vi "T_RH_P.vi"(0 "VISA in":refnum<visa-resource-name>="LuftWS", 5 "WS_Commands":enum16{"OpenWS", "ReadTRHP", "CloseWS"}(ring)=enum."ReadTRHP", 7 "wait (ms)":u32=50, 11 "Error In":errorcluster) -> (4 "VISA out":refnum<visa-resource-name>="LuftWS", 6 "TRHP":T1={"Temp"=27.834401709401718, "RelH"=23.501221001221, "Press"=837.9120879120879, "AbH"=6.333943833943834}, 15 "Error Out":errorcluster)   [LabVIEW 2012]
uses:
  <vilib>/Instr/_visa.llb/VISA Configure Serial Port (Instr).vi
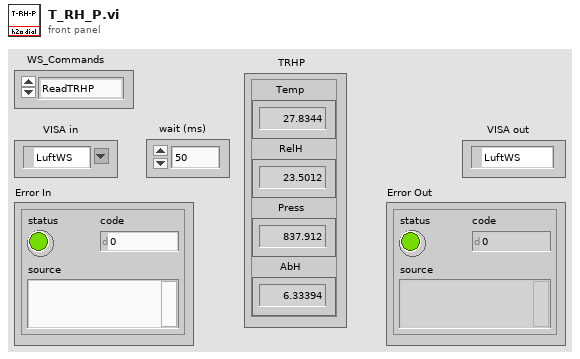
[diagram p1: front panel]
types:
  T1 = cluster{"Temp":dbl, "RelH":dbl, "Press":dbl, "AbH":dbl}
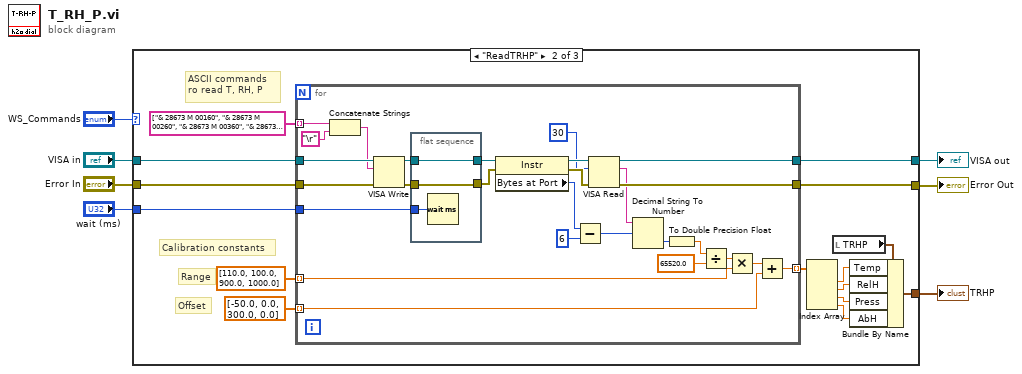
[diagram p0: block diagram]
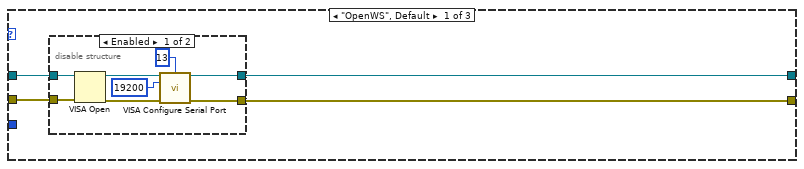
[diagram p2: hidden frame]
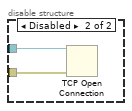
[diagram p3: hidden frame]
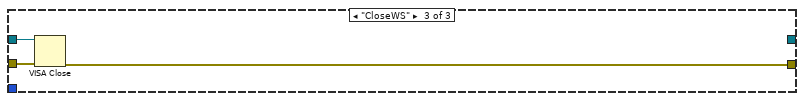
[diagram p4: hidden frame]
diagram:
  n1 = case shown="\"ReadTRHP\"" "WS_Commands" {
    tunnel: "VISA in" -> [w11 w36 w69]
    tunnel: "Error In" -> [w10 w35 w68]
    tunnel: [w9 w33 _] -> w3
    tunnel: [w8 w32 w67] -> w2
    tunnel: "wait (ms)" -> [_ w34 _]
    tunnel: [_ w30 _] -> w1
    frame "OpenWS", Default {
      n2 = disable-structure shown="Enabled" {
        disable-tunnel: w11 -> [w17 w21]
        disable-tunnel: w10 -> [w16 w20]
        disable-tunnel: [w14 _] -> w9
        disable-tunnel: [w13 _] -> w8
        frame Enabled {
          n3 = VISA Open(error in (no error)=w16, VISA resource name=w17) -> (VISA resource name=w19:refnum<visa-resource-name>, error out=w15:errorcluster)  [unwired: 3 in]
          n4 = call-poly "VISA Configure Serial Port"("VISA resource name"=w19, "termination char\n(0xA = '\\n' = LF)"=u8 13 ("termination char\n(0xA = '\\n' = LF)"), "baud rate (9600)"=u32 19200, "error in (no error)"=w15) -> ("VISA resource name out"=w14:refnum<visa-resource-name>, "error out"=w13:errorcluster)  [unwired: 10 in]
        }
        frame Disabled {
          n5 = TCP Open Connection(address=w21, error in (no error)=w20) -> ()  [unwired: 3 in, 2 out]
        }
      }
    }
    frame "ReadTRHP" {
      # "Offset"
      # "Range"
      # "Calibration constants"
      # "ASCII commands\nro read T, RH, P"
      n6 = for {
        tunnel: w36 -> [w63]
        tunnel: w35 -> [w62]
        tunnel: w34 -> [w58]
        tunnel: [w53] -> w33
        tunnel: [w52] -> w32
        tunnel: [w43] -> w26 mode=indexing
        tunnel: string[] ["& 28673 M 00160", "& 28673 M 00260", "& 28673 M 00360", "& 28673 M 00270"] -> [w40] mode=indexing
        tunnel: dbl[] [110.0, 100.0, 900.0, 1000.0] -> [w39] mode=indexing
        tunnel: dbl[] [-50.0, 0.0, 300.0, 0.0] -> [w38] mode=indexing
        n7 = Concatenate Strings(w40, "\r") -> (w59:string)
        n8 = VISA Write(VISA resource name=w63, write buffer=w59, error in (no error)=w62) -> (VISA resource name out=w60:refnum<visa-resource-name>, error out=w61:errorcluster)  [unwired: 1 out]
        n9 = flat-sequence {
          tunnel: [w66] -> w55
          tunnel: w60 -> [w66]
          tunnel: [w65] -> w54
          tunnel: w61 -> [w65]
          tunnel: w58 -> [w64]
          frame #0 {
            n10 = Wait (ms)(milliseconds to wait=w64) -> ()  [unwired: 1 out]
          }
        }
        n11 = property class="Instr"(reference=w55, error in=w54) -> (reference out=w56:refnum<visa-resource-name>, error out=w57:errorcluster, "Bytes at Port"=w51:u32)
        n12 = Subtract(x=w51, y=u32 6) -> (x-y=w48:u32)
        n13 = VISA Read(VISA resource name=w56, byte count=u32 30, error in (no error)=w57) -> (VISA resource name out=w53:refnum<visa-resource-name>, read buffer=w49:string, error out=w52:errorcluster)  [unwired: 1 out]
        n14 = Decimal String To Number(string=w49, offset=w48) -> (number=w47:i32)  [unwired: 1 in, 1 out]
        n15 = To Double Precision Float(number=w47) -> (double precision float=w46:dbl)
        n16 = Divide(x=w46, y=65520.0) -> (x/y=w45:dbl)
        n17 = Multiply(x=w45, y=w39) -> (x*y=w44:dbl)
        n18 = Add(x=w44, y=w38) -> (x+y=w43:dbl)
      }
      n19 = Index Array(array=w26) -> (element #1=w23:dbl, element #2=w24:dbl, element #3=w25:dbl, element #4=w22:dbl)  [unwired: 4 in]
      n20 = local read "TRHP"() -> (w31:T1)
      n21 = Bundle By Name(cluster=w31, "Temp"=w23, "RelH"=w24, "Press"=w25, "AbH"=w22) -> (w30:T1)
    }
    frame "CloseWS" {
      n22 = VISA Close(VISA resource name=w69, error in (no error)=w68) -> (error out=w67:errorcluster)
    }
  }
  "Error Out" <- w2
  "VISA out" <- w3
  "TRHP" <- w1
